vi "Dispose.vi"(8 "error in":errorcluster, 11 "ChicagoPizzaStore":refnum<class "ChicagoPizzaStore.lvclass">) -> (0 "error out":errorcluster)   [LabVIEW 2020, in "FactoryMethod.lvlib" / "PizzaFactoryMethod.lvlib" / "ChicagoPizzaStore.lvclass"]
uses:
  ChicagoPizzaStore.lvclass
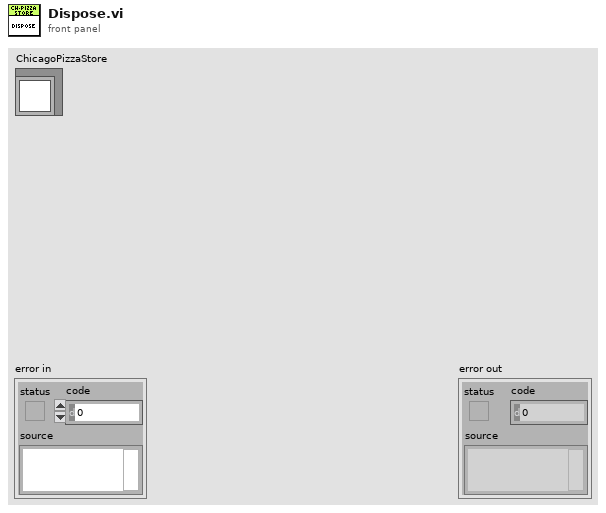
[diagram p1: front panel]
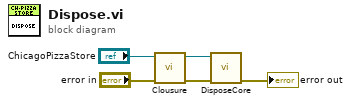
[diagram p0: block diagram]
diagram:
  n1 = call-dynamic "Clousure.vi"("error in (no error)"="error in", "ChicagoPizzaStore"="ChicagoPizzaStore") -> ("error out"=w3:errorcluster, "ChicagoPizzaStore"=w4:refnum<class "ChicagoPizzaStore.lvclass">)  [unwired: 8 in]
  n2 = call-dynamic "DisposeCore.vi"("error in (no error)"=w3, "ChicagoPizzaStore"=w4) -> ("error out"=→"error out":errorcluster)  [unwired: 8 in, 1 out]
